vi "ECG Heart Rate Monitor (Online).vi"() -> ()   [LabVIEW 2023]
doc: "This example simulates a normal ECG signal with and without baseline wandering, in seconds. This example uses the WA Peak Detection VI to extract the peaks and valleys (QRS Complex) of the signal. If the signal contains baseline wandering, select the <b>Detrend</b> option in the <b>Peak Detection Mode</b> control to detrend the signal before extracting the peaks and valleys. This example also shows an application of real-time heart rate extraction, which computes the heart rate from a streaming ECG signal.\n\n<b>Instructions:</b>\n1) Run this VI.\n2) Observe the peaks and valleys of a streaming ECG signal. \n3) Change <b>Simulation Mode </b>and <b>Peak Detection Mode</b> to observe the difference among the results."
uses:
  <vilib>/addons/Wavelet Analysis/online wavelet analysis.llb/WA Online Multiscale Peak Detection (Waveform).vi
  <vilib>/measure/NI_MABase.lvlib
  <vilib>/addons/_Advanced Signal Processing/NI_AdvSigProcOnlineWA.lvlib
panel:
  out "Peak/Valley Plot":cluster{"location":dbl[], "amplitude":dbl[]}[](graph)
  in  "Peak Detecion Mode":enum16{"Detrend", "No Detrend"}(ring)
  in  "Simulation Mode":enum16{"Baseline", "No Baseline"}(ring)
  out "Heart Rate":dbl[](graph)
  in  "stop":bool
  # "Overview: Simulates a normal ECG signal with and without baseline wandering, in seconds. \nRequirements: LabVIEW Full Development System, Advanced Signal Processing Toolkit\nInstructions: \n1. Run this VI.\n2. Observe the peaks and valleys of a streaming ECG signal. \n3. Change Simulation Mode and Peak Detection Mode to observe the difference among the results.\n4. Click Stop to stop the VI."
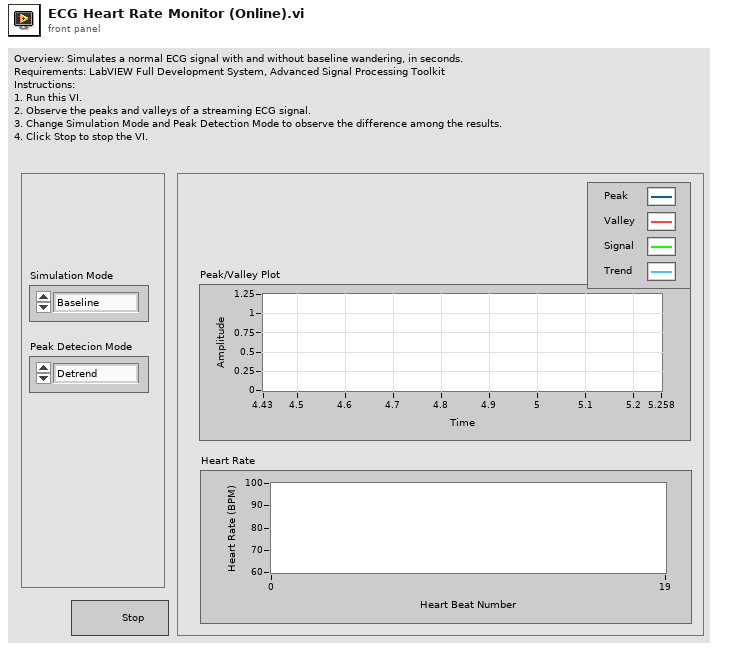
[diagram p1: front panel]
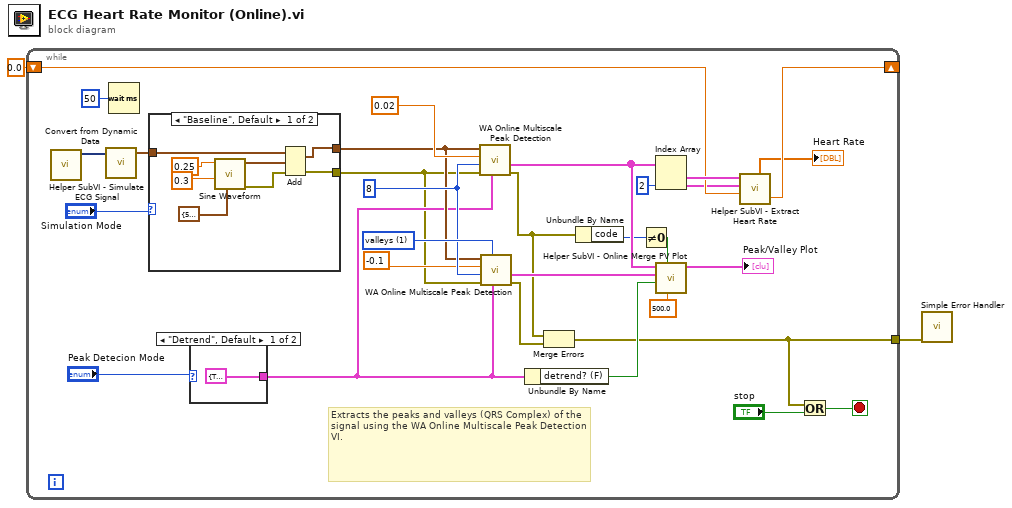
[diagram p0: block diagram]
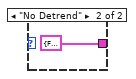
[diagram p3: hidden frame]
diagram:
  n1 = while {
    shift-right: [w24] -> _
    shift-left: 0.0 -> [w25]
    tunnel: [w3] -> w1
    stop <- w4 stop-if-true
    w30 = u16 1 items=["peaks", "valleys"] ("peaks/valleys")
    w29 = 8 ("width")
    # "Extracts the peaks and valleys (QRS Complex) of the signal using the WA Online Multiscale Peak Detection VI."
    n2 = call "Helper SubVI - Simulate ECG Signal.vi"() -> ("Data"=w27:dynamicdata)  [unwired: 11 in]
    n3 = call "Convert from Dynamic Data"("Dynamic Data Type"=w27) -> ("Waveform"=w22:waveform(dbl))  [unwired: 1 in, 2 out]
    n4 = Wait (ms)(milliseconds to wait=u32 50 ("millisecond multiple")) -> ()  [unwired: 1 out]
    n5 = case shown="\"Baseline\", Default" "Simulation Mode" {
      tunnel: w22 -> [w37 w41]
      tunnel: [w35 w41] -> w21
      tunnel: [w33 _] -> w8
      frame "Baseline", Default {
        n6 = call <vilib>:"Sine Waveform.vi"("sampling info"=cluster{"Fs":dbl, "#s":dbl} {"Fs"=500.0, "#s"=500.0}, "amplitude"=0.3, "frequency"=0.25) -> ("error out"=w34:errorcluster, "signal out"=w36:waveform(dbl))  [unwired: 4 in, 3 out]
        n7 = Add(1:w36, 2:w37, 4:w34) -> (0:w35:waveform(dbl), 3:w33:errorcluster)
      }
      frame "No Baseline" {
      }
    }
    n8 = case shown="\"Detrend\", Default" "Peak Detecion Mode" {
      tunnel: [cluster{"detrend? (F)":bool, "trend level":dbl} {"detrend? (F)"=TRUE, "trend level"=0.5} ("detrend settings") cluster{"detrend? (F)":bool, "trend level":dbl} {"detrend? (F)"=FALSE, "trend level"=0.0} ("detrend settings")] -> w14
      frame "Detrend", Default {
      }
      frame "No Detrend" {
      }
    }
    n9 = call-poly <vilib>:"WA Online Multiscale Peak Detection.vi"("detrend settings"=w14, "error in (no error)"=w8, "width"=w29, "threshold"=0.02, "signal"=w21) -> ("error out"=w7:errorcluster, "peak plot"=w16:cluster{"Ramp Pattern":dbl[], "X":dbl[]}[])  [unwired: 3 in, 2 out]
    n10 = call-poly <vilib>:"WA Online Multiscale Peak Detection.vi"("detrend settings"=w14, "peaks/valleys"=w30, "error in (no error)"=w8, "width"=w29, "threshold"=-0.1, "signal"=w21) -> ("error out"=w6:errorcluster, "peak plot"=w15:cluster{"Ramp Pattern":dbl[], "X":dbl[]}[])  [unwired: 2 in, 2 out]
    n11 = Unbundle By Name(w14) -> ("detrend? (F)"=w13:bool)
    n12 = Merge Errors(w7, w6) -> (w3:errorcluster)
    n13 = Unbundle By Name(w7) -> ("code"=w10:i32)
    n14 = Not Equal To 0?(x=w10) -> (x != 0?=w9:bool)
    n15 = Index Array(array=w16, index #2=2 ("index")) -> (element #1=w26:cluster{"Ramp Pattern":dbl[], "X":dbl[]}, element #2=w19:cluster{"Ramp Pattern":dbl[], "X":dbl[]})  [unwired: 1 in]
    n16 = call "Helper SubVI - Online Merge PV Plot.vi"("sampling rate"=500.0, "initialize? (F)"=w9, "trend  (peak:T)"=w13, "valley plot"=w15, "peak plot"=w16) -> ("peak valley plot"=→"Peak/Valley Plot":cluster{"location":dbl[], "amplitude":dbl[]}[])  [unwired: 6 in]
    n17 = call "Helper SubVI - Extract Heart Rate.vi"("last peak"=w25, "trend"=w19, "peaks"=w26) -> ("last peak out"=w24:dbl, "HR"=→"Heart Rate":dbl[])  [unwired: 1 in, 6 out]
    n18 = Or(x=w3, y="stop") -> (x .or. y?=w4:bool)
  }
  n19 = call <vilib>:"Simple Error Handler.vi"("error in (no error)"=w1) -> ()  [unwired: 4 in, 5 out]
